vi "Do.vi"(8 "error in":errorcluster, 10 "Actor in":refnum<class "Actor.lvclass">, 11 "Remove Log Message MSG":refnum<class "Remove Log Message MSG.lvclass">) -> (0 "error out":errorcluster, 2 "Actor out":refnum<class "Actor.lvclass">)   [LabVIEW 2016, in "Controller.lvlib" / "Remove Log Message MSG.lvclass"]
doc: "(<B>Filename</B>: Actor Framework.lvlib:Message.lvclass:Do.vi)\n\nDefines what a message does when it is received by an actor. Generally, a message instructs an actor to invoke one of its methods. By default, this method does nothing. A child class must override it to define behavior. Create a child class by using the Actor Framework Message Maker dialog box."
uses:
  Remove Log Message MSG.lvclass
  <vilib>/ActorFramework/Actor/Actor.lvclass
  gController.lvclass
  Read DataMap.vi
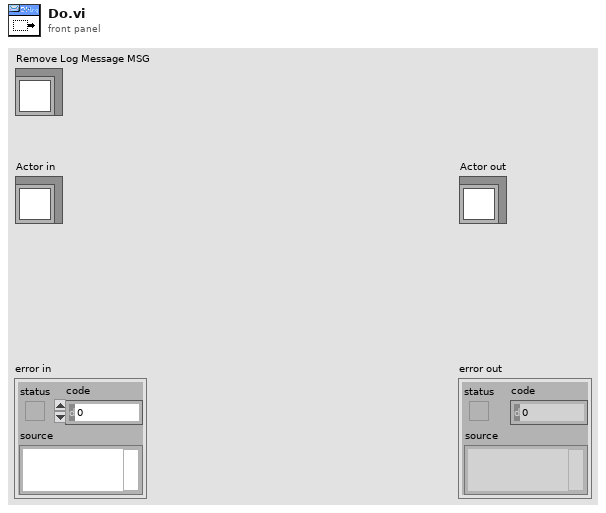
[diagram p1: front panel]
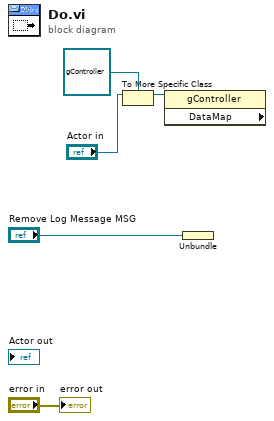
[diagram p0: block diagram]
diagram:
  n1 = To More Specific Class(target class=refnum<class "gController.lvclass"> refnum ("Controller.lvlib:gController"), reference="Actor in") -> (specific class reference=w2:refnum<class "gController.lvclass">)  [unwired: 1 in, 1 out]
  n2 = property class="gController" props=["DataMap"](reference=w2) -> ()  [unwired: 1 in, 3 out]
  n3 = Unbundle("Remove Log Message MSG") -> ()  [unwired: 1 out]
  "error out" <- "error in"
